vi "cozvd.vi"() -> ()   [LabVIEW 2019]
uses:
  <vilib>/platform/TimedLoop/XDataNode/XDataNode.xnode
  <vilib>/Platform/TimedLoop/XDataNode/nitl_modes.ctl
  <vilib>/Platform/TimedLoop/XDataNode/XDNodeRunTimeDep.lvlib
  <vilib>/Platform/TimedLoop/XDataNode/wakeup.ctl
  <vilib>/Platform/TimedLoop/XDataNode/timing_clust.ctl
  <vilib>/myRIO/Express VI/Onboard Devices/Accelerometer/Accelerometer Express VI.xnode
  <vilib>/myRIO/Instrument Drivers/Onboard Devices/Accelerometer/vis/Read.vi
  <vilib>/myRIO/Instrument Drivers/Onboard Devices/Accelerometer/Accelerometer.lvlib
  <vilib>/myRIO/Common/Instrument Driver Framework/myRIO v1.0/Accelerometer/typedefs/Accelerometer Channels Enum.ctl
  <vilib>/myRIO/Common/Instrument Driver Framework/myRIO v1.0/Accelerometer/typedefs/Accelerometer Channels List.ctl
  <vilib>/myRIO/Common/Instrument Driver Framework/Utilities/typedefs/Generic FPGA Reference.ctl
  <vilib>/myRIO/Common/Instrument Driver Framework/Utilities/typedefs/myRIO v1.0 Reference.ctl
  <vilib>/myRIO/Common/Instrument Driver Framework/Utilities/typedefs/Hardware Version Enum.ctl
  <vilib>/myRIO/Common/Instrument Driver Framework/Utilities/typedefs/myRIO Generic Hardware Reference.ctl
  <vilib>/myRIO/Instrument Drivers/Onboard Devices/Accelerometer/typedefs/Accelerometer Reference.ctl
  <vilib>/myRIO/Instrument Drivers/Onboard Devices/Accelerometer/vis/myRIO Accelerometer Open.xnode
  <vilib>/myRIO/Common/Instrument Driver Framework/Utilities/vis/Is FPGA Ref Available.vi
  <vilib>/myRIO/Common/Instrument Driver Framework/myRIO v1.0/Accelerometer/vis/myRIO v1.1 Open Accelerometer.vi
  <vilib>/userDefined/High Color/nirio_resource_hc.ctl
panel:
  out "Vset":dbl
  out "run_time":dbl
  out "vfb":dbl
  out "dec time":dbl
  in  "resetgraph2":bool=TRUE caption="Reset"
  out "duty3":dbl
  out "duty2":dbl
  out "duty1":dbl
  in  "Reset":bool
  out "Y_sp":dbl
  out "X_sp":dbl
  in  "Toa do":dbl[][](array[numeric])
  out "Y_ph":dbl
  out "X_ph":dbl
  out "Map":cluster{"Y":dbl[], "Y":dbl[]}[](graph)
  out "V3_sp":dbl
  out "V3_ph":dbl
  out "Waveform Chart":T1(graph)
  in  "Kd":dbl
  in  "Ki":dbl
  in  "Kp":dbl
  out "V2_ph":dbl
  out "V1_ph":dbl
  out "V2_sp":dbl
  out "V1_sp":dbl
  in  "Start":bool
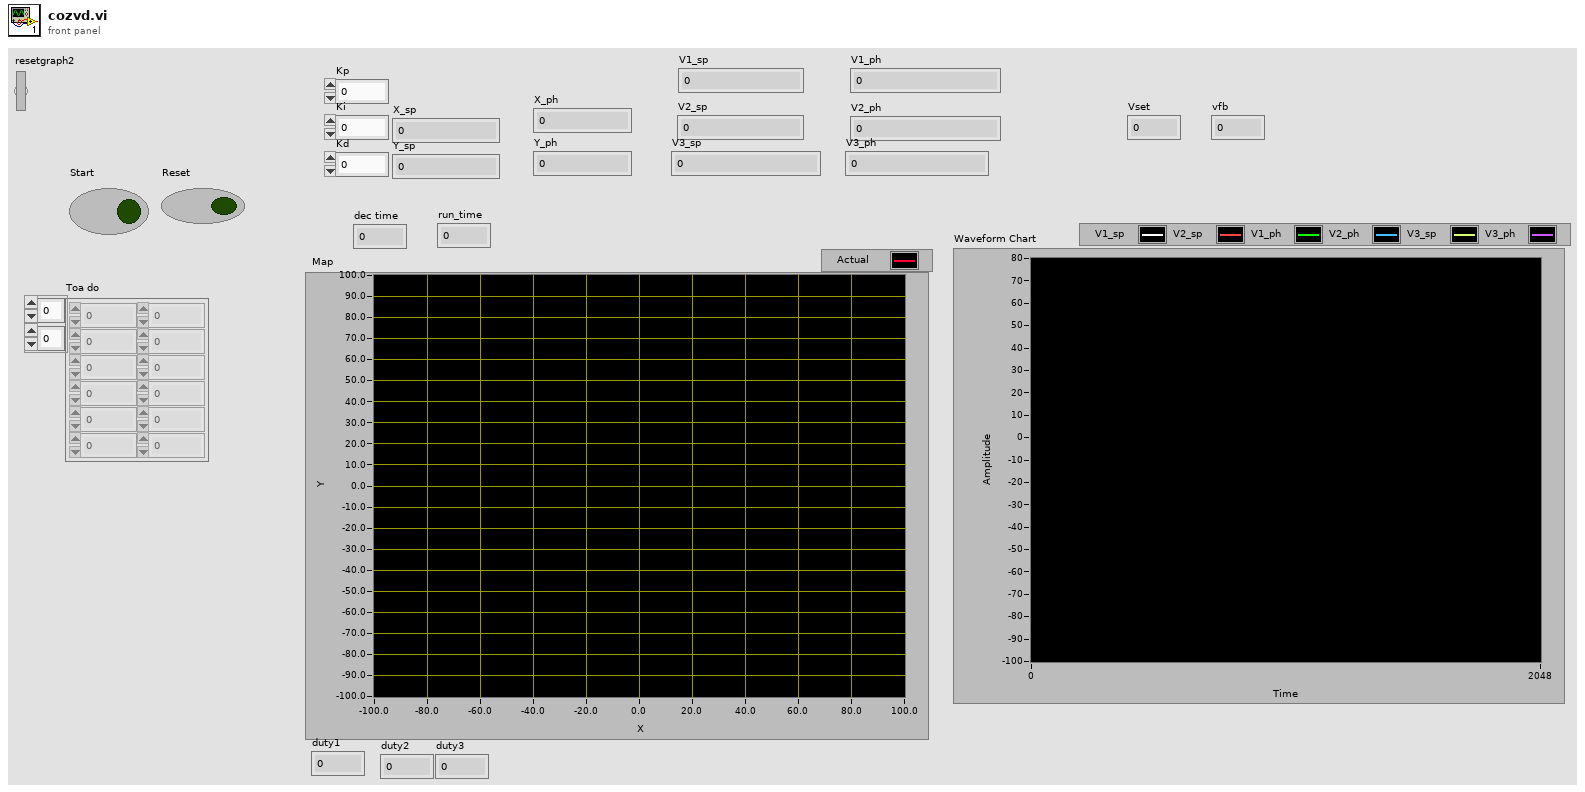
[diagram p1: front panel]
types:
  T1 = cluster{dbl, dbl, "V1_ph":dbl, "V2_ph":dbl, dbl, "V3_ph":dbl}
  T2 = typedef "XDNodeRunTimeDep.lvlib/timing_clust.ctl" = cluster{"Expected End [f-1]":u64, "Actual End [f-1]":u64, "Finished Late? [f-1]":bool, "Expected End [i-1]":u64, "Actual End [i-1]":u64, "Finished Late? [i-1]":bool, "Expected Start [i]":u64, "Actual Start [i]":u64, "Expected Start [f]":u64, "Actual Start [f]":u64, "Source Name":string, "Structure Name":string, "Period":i64, "Deadline":i64, "Offset":i64, "Start":i64, "Priority":i32, "Timeout":i32, "Mode":T3, "Wakeup Reason":T4, "Error":errorcluster, "Source Type":string, "Secondary Source Type":string, "Global End Time":u64, "Global Start Time":u64, "Frame Duration":u64, "Iteration Duration":u64, "Assigned CPU":i32, "I/O Scan Engine Mode":u32}
  T3 = typedef "XDNodeRunTimeDep.lvlib/nitl_modes.ctl" = enum32{"No Change", "Process missed periods, maintain original phase", "Discard missed periods, maintain original phase", "Process missed periods, ignore original phase", "Discard missed periods, ignore original phase"}
  T4 = typedef "XDNodeRunTimeDep.lvlib/wakeup.ctl" = enum32{"Normal", "Aborted", "Asynchronous wakeup", "Timing source error", "Timed loop error", "Timeout"}
  T5 = typedef "Accelerometer.lvlib/Accelerometer Reference.ctl" = cluster{"myRIO Reference":T6, "Accelerometer Channels List":T10, "LSB Weight":dbl}
  T6 = typedef "myRIO Generic Hardware Reference.ctl" = cluster{"myRIO Model":T7, "myRIO Hardware Reference":T8}
  T7 = typedef "Hardware Version Enum.ctl" = enum16{"Unknown", "myRIO-1900", "myRIO-1950", "roboRIO", "NI ELVIS RIO CM", "ELVIS III"}
  T8 = typedef "myRIO v1.0 Reference.ctl" = cluster{"Generic FPGA Reference":T9, "Allow multiple opens":bool}
  T9 = typedef "Generic FPGA Reference.ctl" = refnum<k20>
  T10 = typedef "Accelerometer Channels List.ctl" = T11[]
  T11 = typedef "Accelerometer Channels Enum.ctl" = enum16{"Not Connected", "X-Axis", "Y-Axis", "Z-Axis"}
  T12 = typedef "nirio_resource_hc.ctl" = tag
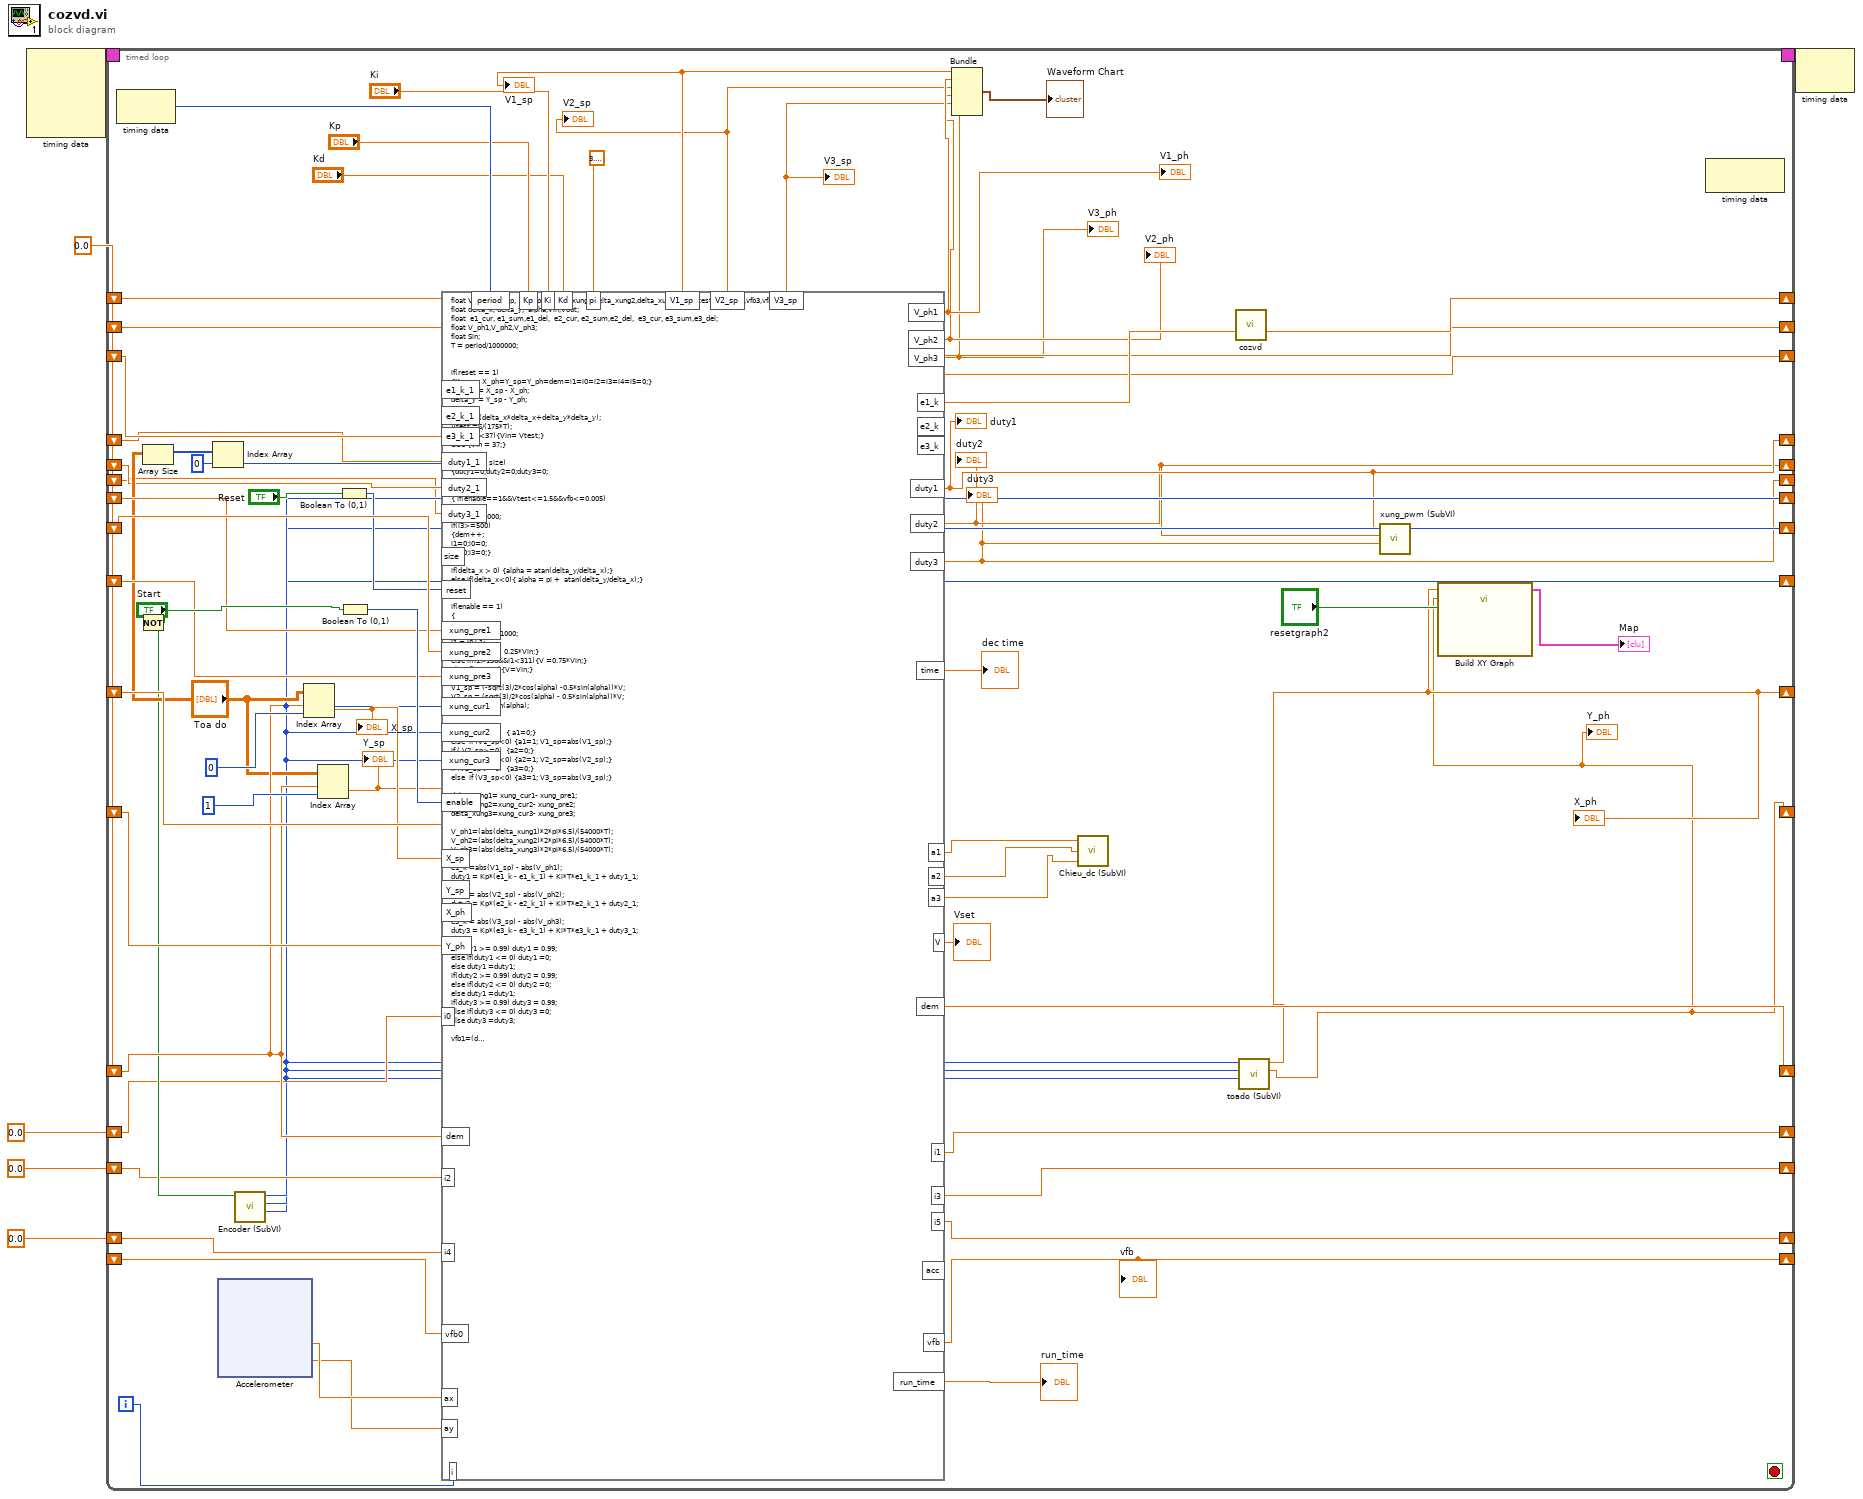
[diagram p0: block diagram]
diagram:
  w4 = 0.0 ("e1")
  n1 = node-c288() -> (w6:T2)  [unwired: 4 in]
  n2 = timed-loop {
    timing: w6 -> [_]
    timing-out: [_] -> w5
    shift-right: [w74] -> _
    shift-left: w4 -> [w72]
    shift-right: [w73] -> _
    shift-left: w4 -> [w71]
    shift-right: [w25] -> _
    shift-left: w4 -> [w59]
    shift-right: [w24] -> _
    shift-left: w4 -> [w68]
    shift-right: [w62] -> _
    shift-left: w4 -> [w61]
    shift-right: [w23] -> _
    shift-left: w4 -> [w60]
    shift-right: [w22] -> _
    shift-left: w4 -> [w58]
    shift-right: [w21] -> _
    shift-left: w4 -> [w57]
    shift-right: [w54] -> _
    shift-left: w4 -> [w53]
    shift-right: [w19] -> _
    shift-left: _ -> [w34]
    shift-right: [w30] -> _
    shift-left: 0.0 ("i1") -> [w29]
    shift-right: [w28] -> _
    shift-left: 0.0 ("i3") -> [w27]
    shift-right: [w18] -> _
    shift-left: 0.0 ("i5") -> [w20]
    shift-right: [w12] -> _
    shift-left: _ -> [w15]
    shift-right: [w11] -> _
    shift-left: _ -> [w14]
    shift-right: [w10] -> _
    shift-left: _ -> [w13]
    i -> [w33]
    stop <- _ stop-if-true
    n3 = node-c288() -> (w67:i64)  [unwired: 1 in]
    n4 = Not(x="Start") -> (.not. x?=w35:bool)
    n5 = Array Size(array="Toa do") -> (size(s)=w48:i32[])
    n6 = Index Array(array=w48, index=0) -> (element=w46:i32)
    n7 = xnode "Accelerometer"() -> ("X-Axis"=w32:dbl, "Y-Axis"=w31:dbl)  [unwired: 1 in, 1 out]
    n8 = call "Encoder (SubVI).vi"("Boolean"=w35) -> ("Counter Value3"=w23:i32, "Counter Value 2"=w24:i32, "Counter Value"=w25:i32)  [unwired: 8 in]
    n9 = Index Array(array="Toa do", index (row)=w53, index (col)=0 ("disabled index (col)")) -> (element=w51:dbl)
    "X_sp" <- w51
    n10 = Index Array(array="Toa do", index (row)=w53, index (col)=1 ("disabled index (col)")) -> (element=w50:dbl)
    "Y_sp" <- w50
    n11 = Boolean To (0,1)(Boolean="Reset") -> (0, 1=w45:i16)
    n12 = Boolean To (0,1)(Boolean="Start") -> (0, 1=w70:i16)
    n13 = formula code="float V1_sp, V2_sp,  V3_sp,T, delta_xung1,delta_xung2,delta_xung3,V,S,Vtest,vfb1,vfb2,vfb3,vfb,acc;\nfloat delta_x, delta_y,  alpha,Vin,Vout;\nfloat  e1_cur, e1_sum,e1_del,  e2_cur, e2_sum,e2_del,  e3_cur, e3_sum,e3_del;\nfloat V_ph1,V_ph2,V_ph3;\nfloat Sin;\nT = period/1000000;\n\n\nif(reset == 1)\n{X_sp = X_ph=Y_sp=Y_ph=dem=i1=i0=i2=i3=i4=i5=0;}\ndelta_x = X_sp - X_ph;\ndelta_y = Y_sp - Y_ph;\n\nS = sqrt(delta_x*delta_x+delta_y*delta_y); \nVtest =S/(175*T);\nif(Vtest <37){Vin= Vtest;}\nelse {Vin = 37;}\n\nif(dem == size)\n{duty1=0;duty2=0;duty3=0;\ni5 = i4;}\nelse\n{ if(enable==1&&Vtest<=1.5&&vfb<=0.005)\n i3=i2+1;\ntime =i3/1000;\nif(i3>=500)\n{dem++;\ni1=0;i0=0;\ni2=0;i3=0;}\n\nif(delta_x > 0) {alpha = atan(delta_y/delta_x);}\nelse if(delta_x<0){ alpha = pi +  atan(delta_y/delta_x);}\n\n\nif(enable == 1)\n{\ni5=i4+1;\nrun_time = i5/1000;\ni1 = i0+1;\nif(i1<156){V = 0.25*Vin;}\nelse if(i1>156&&i1<311){V =0.75*Vin;}\nelse if(i1>311){V=Vin;}\n\nV1_sp = (-sqrt(3)/2*cos(alpha) -0.5*sin(alpha))*V;\nV2_sp = (sqrt(3)/2*cos(alpha) - 0.5*sin(alpha))*V;\n V3_sp = V*sin(alpha); \n\n\nif ( V1_sp>=0)  { a1=0;}\nelse  if (V1_sp<0) {a1=1; V1_sp=abs(V1_sp);}\nif ( V2_sp>=0)  {a2=0;}\nelse  if (V2_sp<0) {a2=1; V2_sp=abs(V2_sp);}\nif (V3_sp >=0)  {a3=0;}\nelse  if (V3_sp<0) {a3=1; V3_sp=abs(V3_sp);}\n\ndelta_xung1= xung_cur1- xung_pre1;\ndelta_xung2=xung_cur2- xung_pre2;\ndelta_xung3=xung_cur3- xung_pre3; \n\nV_ph1=(abs(delta_xung1)*2*pi*6.5)/(54000*T);\nV_ph2=(abs(delta_xung2)*2*pi*6.5)/(54000*T);\nV_ph3=(abs(delta_xung3)*2*pi*6.5)/(54000*T);\n\ne1_k =abs(V1_sp) - abs(V_ph1);\nduty1 = Kp*(e1_k - e1_k_1) + Ki*T*e1_k_1 + duty1_1;\n\ne2_k = abs(V2_sp) - abs(V_ph2);\nduty2 = Kp*(e2_k - e2_k_1) + Ki*T*e2_k_1 + duty2_1;\n\ne3_k = abs(V3_sp) - abs(V_ph3);\nduty3 = Kp*(e3_k - e3_k_1) + Ki*T*e3_k_1 + duty3_1;\n\nif(duty1 >= 0.99) duty1 = 0.99;\nelse if(duty1 <= 0) duty1 =0;\nelse duty1 =duty1;\nif(duty2 >= 0.99) duty2 = 0.99;\nelse if(duty2 <= 0) duty2 =0;\nelse duty1 =duty1;\nif(duty3 >= 0.99) duty3 = 0.99;\nelse if(duty3 <= 0) duty3 =0;\nelse duty3 =duty3;\n\nvfb1=(delta_xung1)*2*pi*6.5/(54000*T);\nvfb2=(delta_xung2)*2*pi*6.5/(54000*T);\nvfb3=(delta_xung3)*2*pi*6.5/(54000*T);\nvfb = sqrt(1/3*(vfb1-vfb2)*(vfb1-vfb2)+vfb3*vfb3);\nacc = sqrt(ax*ax+ay*ay);\n}\n}"("Kp"="Kp", "Ki"="Ki", "Kd"="Kd", "pi"=3.141592653589793, "e1_k_1"=w72, "e2_k_1"=w71, "xung_pre1"=w59, "xung_pre2"=w68, "xung_cur1"=w25, "xung_cur2"=w24, "enable"=w70, "period"=w67, "e3_k_1"=w61, "xung_cur3"=w23, "xung_pre3"=w60, "X_ph"=w58, "X_sp"=w51, "Y_sp"=w50, "Y_ph"=w57, "dem"=w53, "size"=w46, "reset"=w45, "i"=w33, "vfb0"=w34, "ax"=w32, "ay"=w31, "i0"=w29, "i2"=w27, "i4"=w20, "duty1_1"=w15, "duty2_1"=w14, "duty3_1"=w13) -> ("V1_sp"=w43:dbl, "V_ph1"=w42:dbl, "V_ph2"=w40:dbl, "e1_k"=w74:dbl, "e2_k"=w73:dbl, "V2_sp"=w41:dbl, "duty1"=w12:dbl, "duty2"=w11:dbl, "e3_k"=w62:dbl, "V_ph3"=w39:dbl, "V3_sp"=w38:dbl, "duty3"=w10:dbl, "a1"=w9:dbl, "a2"=w8:dbl, "a3"=w7:dbl, "dem"=w54:dbl, "vfb"=w19:dbl, "i1"=w30:dbl, "i3"=w28:dbl, "time"=→"dec time":dbl, "i5"=w18:dbl, "run_time"=→"run_time":dbl, "V"=→"Vset":dbl)  [unwired: 1 out]
    "V1_sp" <- w43
    "V2_sp" <- w41
    "V1_ph" <- w42
    "V2_ph" <- w40
    "V3_ph" <- w39
    "V3_sp" <- w38
    "duty1" <- w12
    "duty2" <- w11
    "duty3" <- w10
    "vfb" <- w19
    n14 = Bundle(w43, w42, w41, w40, w38, w39) -> (→"Waveform Chart":cluster{dbl, dbl, dbl, dbl, dbl, dbl})  [unwired: 1 in]
    n15 = call "Chieu_dc (SubVI).vi"("a3"=w7, "a2"=w8, "a1"=w9) -> ()
    n16 = call "cozvd.vi"() -> ()  [unwired: 12 in]
    n17 = call "toado (SubVI).vi"("X3"=w23, "X2"=w24, "X1"=w25) -> ("Y_ph"=w21:dbl, "X_ph"=w22:dbl)  [unwired: 7 in]
    "X_ph" <- w22
    "Y_ph" <- w21
    n18 = call "xung_pwm (SubVI).vi"("duty3 in"=w10, "duty2 in"=w11, "duty1 in"=w12) -> ()  [unwired: 6 in, 3 out]
    n19 = call "Build XY Graph"("Reset"="resetgraph2", "Y Input"=w21, "X Input"=w22) -> ("XY Graph"=→"Map":cluster{"X":dbl[], "Y":dbl[]}[])  [unwired: 7 in, 1 out]
    n20 = node-c288() -> ()  [unwired: 1 in, 1 out]
  }
  n21 = node-c288(w5) -> ()  [unwired: 1 out]
